vi "Convert_CSV_File_to_2D_String_Array.vi"(8 "error in":errorcluster, 11 "CSV File Path":path=path "R:/Manufacturing/Test Engineering/TE_Working/TPS/BOS/SWORDS/wikipedia example.txt") -> (0 "error out":errorcluster, 2 "2-D Array":string[][](table), 3 "Path out":path)   [LabVIEW 2015]
doc: "<b>http://en.wikipedia.org/wiki/Comma-separated_values</b>\n\nReads a CSV formatted text file into a 2D array of strings. The LabVIEW standard Read from Spreadsheet File VI does not support escaped commas or fields that contain CR or LF elements as outlined in RFC 4180\n\nRev 0.0.0 05/09/2011 P. Brooks\n Originated."
panel:
  # "http://en.wikipedia.org/wiki/Comma-separated_values"
  # "http://tools.ietf.org/html/rfc4180"
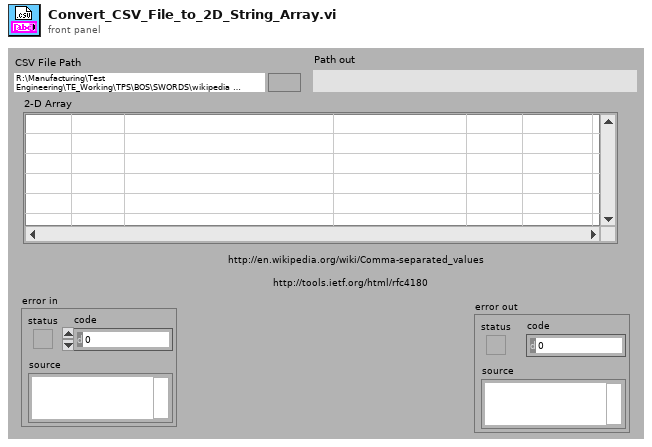
[diagram p1: front panel]
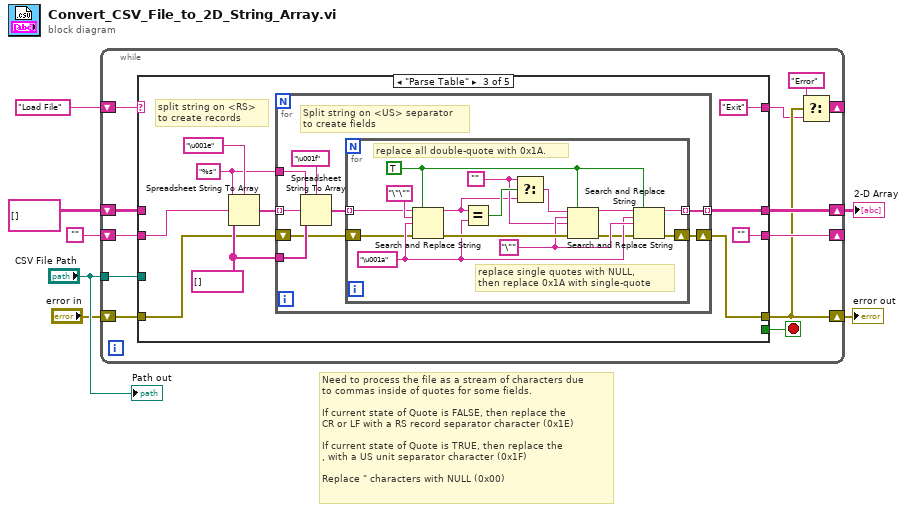
[diagram p0: block diagram]
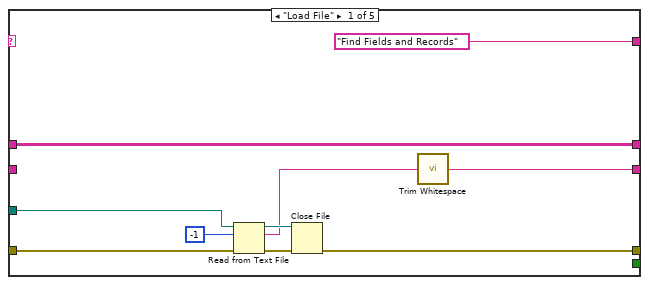
[diagram p2: hidden frame]
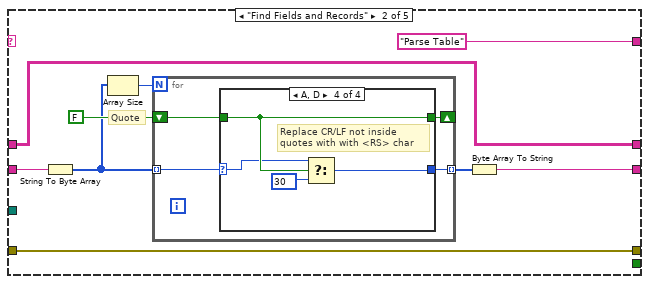
[diagram p3: hidden frame]
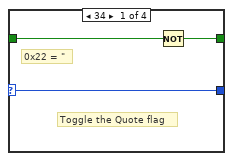
[diagram p4: hidden frame]
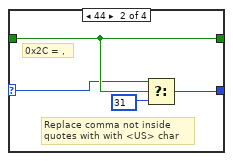
[diagram p5: hidden frame]
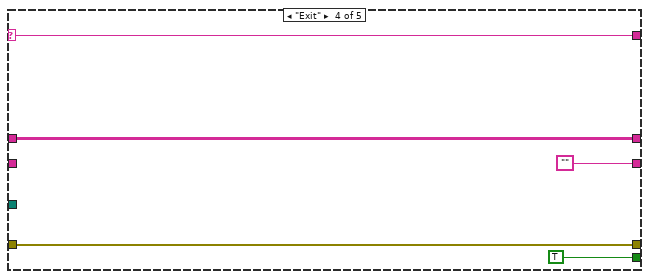
[diagram p7: hidden frame]
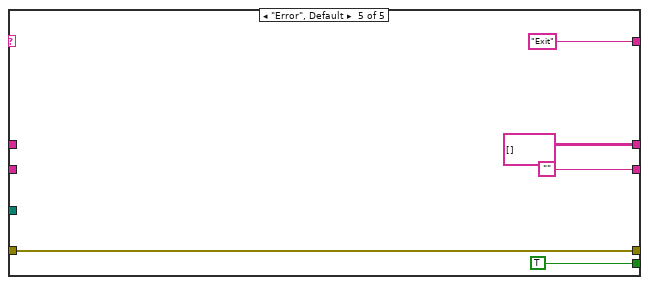
[diagram p8: hidden frame]
diagram:
  # "Need to process the file as a stream of characters due \nto commas inside of quotes for some fields.\n\nIf current state of Quote is FALSE, then replace the\nCR or LF with a RS record separator character (0x1E)\n\nIf current state of Quote is TRUE, then replace the\n, with a US unit separator character (0x1F)\n\nReplace \" characters with NULL (0x00)"
  n1 = while {
    tunnel: "CSV File Path" -> [w18]
    shift-right: [w19] -> _
    shift-left: "" -> [w17]
    shift-right: [w9] -> _
    shift-left: "Load File" -> [w14]
    shift-right: [w16] -> w1
    shift-left: string[][] [] -> [w15]
    shift-right: [w12] -> w2
    shift-left: "error in" -> [w13]
    stop <- w8 stop-if-true
    n2 = case shown="\"Parse Table\"" w14 {
      selector: w14 -> [_ _ _ w92 _]
      tunnel: [w20 w33 "" "" ""] -> w19
      tunnel: w18 -> [w25 _ _ _ _]
      tunnel: ["Find Fields and Records" "Parse Table" "Exit" ("t") w92 "Exit" ("t")] -> w11
      tunnel: [_ _ _ TRUE TRUE] -> w8
      tunnel: w17 -> [_ w31 w57 _ _]
      tunnel: [w26 w32 w62 w89 string[][] []] -> w16
      tunnel: w15 -> [w26 w32 _ w89 _]
      tunnel: [w29 w30 w59 w93 w98] -> w12
      tunnel: w13 -> [w28 w30 w56 w93 w98]
      frame "Load File" {
        n3 = Read from Text File(file (use dialog)=w25, count=-1, error in=w28) -> (refnum out=w24:refnum<file>, text=w21:string, error out=w22:errorcluster)  [unwired: 2 out]
        n4 = Close File(refnum=w24, error in=w22) -> (error out=w29:errorcluster)  [unwired: 1 out]
        n5 = call <vilib>:"Trim Whitespace.vi"("string"=w21) -> ("trimmed string"=w20:string)  [unwired: 1 in]
      }
      frame "Find Fields and Records" {
        # "Quote"
        n6 = String To Byte Array(string=w31) -> (unsigned byte array=w36:u8[])
        n7 = Array Size(array=w36) -> (size(s)=w37:i32)
        n8 = for {
          N: w37 -> [_]
          tunnel: w36 -> [w39] mode=indexing
          shift-right: [w41] -> _
          shift-left: FALSE -> [w42]
          tunnel: [w40] -> w34 mode=indexing
          n9 = case shown="A, D" w39 {
            selector: w39 -> [w44 w48 w50 w52]
            tunnel: w42 -> [w43 w49 w51 w55]
            tunnel: [w45 w49 w51 w55] -> w41
            tunnel: [w44 w46 w50 w53] -> w40
            frame 34 {
              # "0x22 = \""
              # "Toggle the Quote flag"
              n10 = Not(x=w43) -> (.not. x?=w45:bool)
            }
            frame 44 {
              # "0x2C = ,"
              # "Replace comma not inside \nquotes with with <US> char"
              n11 = Select(t=w48, s=w49, f=u8 31) -> (s? t:f=w46:u8)
            }
            frame 0, Default {
            }
            frame 10, 13 {
              # "Replace CR/LF not inside \nquotes with with <RS> char"
              n12 = Select(t=w52, s=w55, f=u8 30) -> (s? t:f=w53:u8)
            }
          }
        }
        n13 = Byte Array To String(unsigned byte array=w34) -> (string=w33:string)
      }
      frame "Parse Table" {
        w65 = string[] []
        w60 = "%s" ("format string")
        # "split string on <RS>\nto create records"
        n14 = Spreadsheet String To Array(delimiter (Tab)="\u001e", format string=w60, spreadsheet string=w57, array type (2D Dbl)=w65) -> (array=w64:string[])
        n15 = for {
          tunnel: w64 -> [w73] mode=indexing
          tunnel: w65 -> [w70]
          tunnel: [w69] -> w62 mode=indexing
          tunnel: w60 -> [w68]
          shift-right: [w66] -> w59
          shift-left: w56 -> [w67]
          # "Split string on <US> separator\nto create fields"
          n16 = Spreadsheet String To Array(delimiter (Tab)="\u001f", format string=w68, spreadsheet string=w73, array type (2D Dbl)=w70) -> (array=w71:string[])
          n17 = for {
            tunnel: w71 -> [w74] mode=indexing
            tunnel: [w75] -> w69 mode=indexing
            shift-right: [w76] -> w66
            shift-left: w67 -> [w78]
            w81 = ""
            w84 = "\"" ("input string")
            w85 = TRUE ("replace all? (F)")
            w83 = "\u001a" ("replace string (\"\")")
            # "replace single quotes with NULL,\nthen replace 0x1A with single-quote"
            # "replace all double-quote with 0x1A."
            n18 = Search and Replace String(replace all?=w85, input string=w74, search string="\"\"", replace string=w83, error in=w78) -> (result string=w80:string, error out=w87:errorcluster)  [unwired: 5 out]
            n19 = Equal?(x=w80, y=w83) -> (x = y?=w82:bool)
            n20 = Select(t=w81, s=w82, f=w80) -> (s? t:f=w79:string)
            n21 = Search and Replace String(replace all?=w85, input string=w79, search string=w84, replace string=w81, error in=w87) -> (result string=w86:string, error out=w77:errorcluster)  [unwired: 5 out]
            n22 = Search and Replace String(replace all?=w85, input string=w86, search string=w83, replace string=w84, error in=w77) -> (result string=w75:string, error out=w76:errorcluster)  [unwired: 1 in, 4 out]
          }
        }
      }
      frame "Exit" {
      }
      frame "Error", Default {
      }
    }
    n23 = Select(t="Error", s=w12, f=w11) -> (s? t:f=w9:string)
  }
  "error out" <- w2
  "2-D Array" <- w1
  "Path out" <- "CSV File Path"
